vi "Configure C-Series Stuff.vi"(8 "error in (no error)":errorcluster, 11 "NI-9239 in":refnum<class "NI-9239 (C Series).lvclass">) -> (0 "error out":errorcluster, 3 "NI-9239 out":refnum<class "NI-9239 (C Series).lvclass">)   [LabVIEW 2020, in "NI-9239 (C Series).lvclass"]
uses:
  NI-9239 (C Series).lvclass
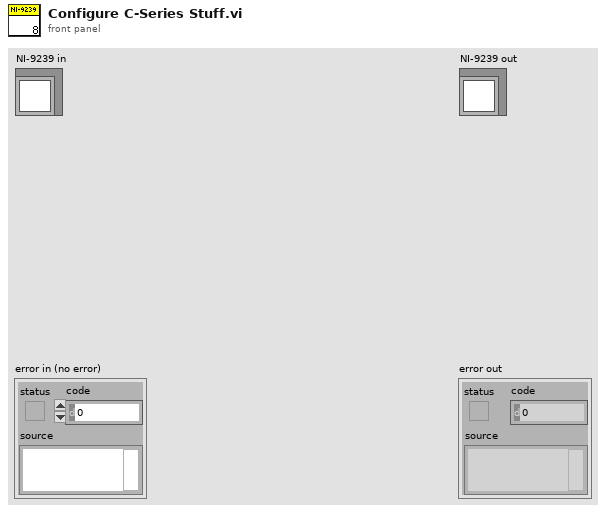
[diagram p1: front panel]
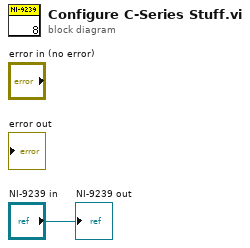
[diagram p0: block diagram]
diagram:
  "NI-9239 out" <- "NI-9239 in"
